vi "detect_edges.vi"() -> ()   [LabVIEW 2019]
uses:
  <vilib>/vision/Image Controls.llb/IMAQ Image.ctl
  <vilib>/vision/NI_Vision_Development_Module.lvlib
panel:
  out "Threshold Range Out":cluster{"Lower value":sgl, "Upper value":sgl}={"Lower value"=128.0, "Upper value"=255.0} {"Upper value" format="%.2f"; "Lower value" format="%.2f"}
  out "Image":T1(plugin-control)
  out "Image Dst Out":T1
  out "Error Out":errorcluster
  in  "Error In":errorcluster
  in  "Sample":string
  in  "File Path":path
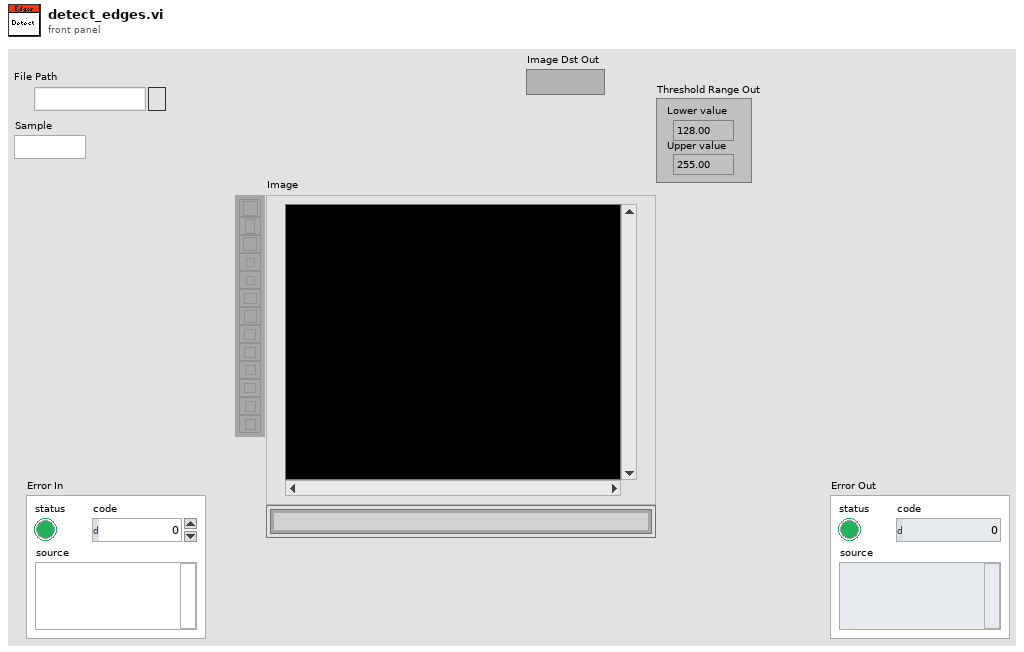
[diagram p1: front panel]
types:
  T1 = typedef "IMAQ Image.ctl" = refnum<image>
  T2 = typedef "Image Type" = u32
  T3 = enum32{"Differentiation", "Gradient", "Prewitt", "Roberts", "Sigma", "Sobel"}
  T4 = enum32{"AutoM", "Close", "Dilate", "Erode", "Gradient", "Gradient in", "Gradient out", "HitMiss", "Open", "PClose", "POpen", "Thick", "Thin"}
  T5 = cluster{"histogram":u32[], "Minimal Value":sgl, "Maximal Value":sgl, "Starting Value":sgl, "Interval Width":sgl, "Mean Value":sgl, "Standard  Variation":sgl, "Area (pixels)":i32}
  T6 = typedef "ROI Descriptor" = cluster{"Global Rectangle":i32[], "Contours":cluster{"ID":enum32{"External", "Internal"}, "Type":u32, "Coordinates":i32[]}[]}
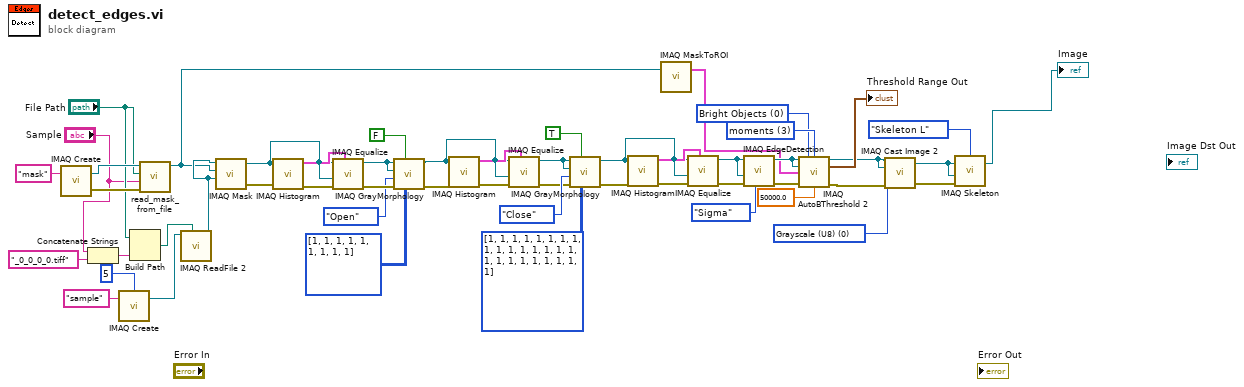
[diagram p0: block diagram]
diagram:
  w7 = T2 0 items=["Grayscale (U8)", "Grayscale (I16)", "Grayscale (SGL)", "Complex (CSG)", "RGB (U32)", "HSL (U32)", "RGB (U64)", "Grayscale (U16)"] ("Image Type")
  w11 = u32 0 items=["Bright Objects", "Dark Objects"] ("Look For (Bright Objects)")
  w14 = 3 items=["clustering", "entropy", "metric", "moments", "inter-class variance"] ("Method (clustering)")
  n1 = call "IMAQ Create"("Image Name"="mask") -> ("New Image"=w26:T1, "error out"=w27:errorcluster)  [unwired: 4 in]
  n2 = Concatenate Strings("Sample", "_0_0_0_0.tiff" ("string")) -> (w24:string)
  n3 = call "IMAQ Create"("Border Size"=5, "Image Name"="sample") -> ("New Image"=w19:T1)  [unwired: 3 in, 1 out]
  n4 = Build Path(base path="File Path", name or relative path=w24) -> (appended path=w21:path)
  n5 = call "read_mask_from_file.vi"("Error In"=w27, "Sample"="Sample", "File Path"="File Path", "Image"=w26) -> ("Image Out"=w13:T1)  [unwired: 5 in, 2 out]
  n6 = call "IMAQ ReadFile 2"("File Path"=w21, "Image"=w19) -> ("Image Out"=w18:T1)  [unwired: 5 in, 4 out]
  n7 = call "IMAQ Mask"("Image Dst"=w18, "Image Mask"=w13, "Image Src"=w18) -> ("error out"=w52:errorcluster, "Image Dst Out"=w17:T1)  [unwired: 2 in]
  n8 = call "IMAQ Histogram"("error in (no error)"=w52, "Image"=w17) -> ("error out"=w51:errorcluster, "Histogram Report"=w50:T5)  [unwired: 8 in]
  n9 = call "IMAQ Equalize"("Histogram Report"=w50, "error in (no error)"=w51, "Image Dst"=w17, "Image Src"=w17) -> ("error out"=w49:errorcluster, "Image Dst Out"=w48:T1)  [unwired: 6 in]
  n10 = call "IMAQ GrayMorphology"("Structuring Element"=i32[][] [[1, 1, 1], [1, 1, 1], [1, 1, 1]], "Square/Hexa (Square)"=FALSE, "error in (no error)"=w49, "Operation"=T4."Open", "Image Dst"=w48, "Image Src"=w48) -> ("error out"=w36:errorcluster, "Image Dst Out"=w37:T1)  [unwired: 4 in]
  n11 = call "IMAQ Histogram"("error in (no error)"=w36, "Image"=w37) -> ("error out"=w38:errorcluster, "Histogram Report"=w39:T5)  [unwired: 8 in]
  n12 = call "IMAQ Equalize"("Histogram Report"=w39, "error in (no error)"=w38, "Image Dst"=w37, "Image Src"=w37) -> ("error out"=w40:errorcluster, "Image Dst Out"=w41:T1)  [unwired: 6 in]
  n13 = call "IMAQ GrayMorphology"("Structuring Element"=i32[][] [[1, 1, 1, 1, 1], [1, 1, 1, 1, 1], [1, 1, 1, 1, 1], [1, 1, 1, 1, 1], [1, 1, 1, 1, 1]], "Square/Hexa (Square)"=TRUE, "error in (no error)"=w40, "Operation"=T4."Close", "Image Dst"=w41, "Image Src"=w41) -> ("error out"=w32:errorcluster, "Image Dst Out"=w33:T1)  [unwired: 4 in]
  n14 = call "IMAQ Histogram"("error in (no error)"=w32, "Image"=w33) -> ("error out"=w35:errorcluster, "Histogram Report"=w34:T5)  [unwired: 8 in]
  n15 = call "IMAQ MaskToROI"("Image"=w13) -> ("ROI Descriptor"=w12:T6)  [unwired: 6 in, 2 out]
  n16 = call "IMAQ Equalize"("Histogram Report"=w34, "error in (no error)"=w35, "Image Dst"=w33, "Image Src"=w33) -> ("error out"=w31:errorcluster, "Image Dst Out"=w30:T1)  [unwired: 6 in]
  n17 = call "IMAQ EdgeDetection"("Method"=T3."Sigma", "error in (no error)"=w31, "Image Dst"=w30, "Image Src"=w30) -> ("error out"=w16:errorcluster, "Image Dst Out"=w15:T1)  [unwired: 6 in]
  n18 = call "IMAQ AutoBThreshold 2"("Image Src"=w15, "Look For (Bright Objects)"=w11, "Method (clustering)"=w14, "Image Dst"=w15, "ROI Descriptor"=w12, "error in (no error)"=w16, "Replace Value (1)"=sgl 50000.0) -> ("Image Dst Out"=w6:T1, "Threshold Range Out"=→"Threshold Range Out":cluster{"Lower value":sgl, "Upper value":sgl}, "error out"=w2:errorcluster)  [unwired: 6 in]
  n19 = call "IMAQ Cast Image 2"("Image Src"=w6, "Image Dst"=w6, "Image Type"=w7, "error in (no error)"=w2) -> ("Image Dst Out"=w5:T1, "error out"=w3:errorcluster)  [unwired: 10 in]
  n20 = call "IMAQ Skeleton"("error in (no error)"=w3, "Image Dst"=w5, "Image Src"=w5, "Mode"=enum32{"Skeleton L", "Skeleton M", "Skiz"}."Skeleton L") -> ("Image Dst Out"=→"Image":T1)  [unwired: 2 in, 1 out]
